vi "Center speed graph cursor on X.vi"(8 "error in (no error)":errorcluster) -> (0 "error out":errorcluster)   [LabVIEW 2020]
uses:
  Globals/gl_Time series viewer globals.vi
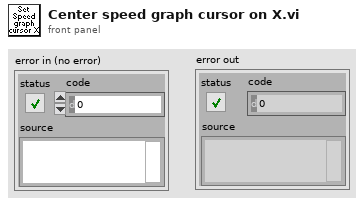
[diagram p1: front panel]
types:
  T1 = typedef "Time series viewer refs.ctl" = cluster{"This VI":refnum<vi>, "Image control":refnum<vi>, "AVI Mode ind":refnum<vi>, "Play":refnum<vi>, "Stop":refnum<vi>, "Back":refnum<vi>, "Scrollbar":refnum<vi>, "Video length info":refnum<vi>, "Expected speed values":refnum<vi>, "Intensity":refnum<vi>, "Path":refnum<vi>, "Selection sliders":refnum<vi>, "Speed Graph ref":refnum<vi>, "Frame rate set (fps)":refnum<vi>, "Number of rows to generate":refnum<vi>, "VL Image Array":refnum<vi>, "Image Scrollbar":refnum<vi>, "Channel to load":refnum<vi>, "Colour":refnum<vi>}
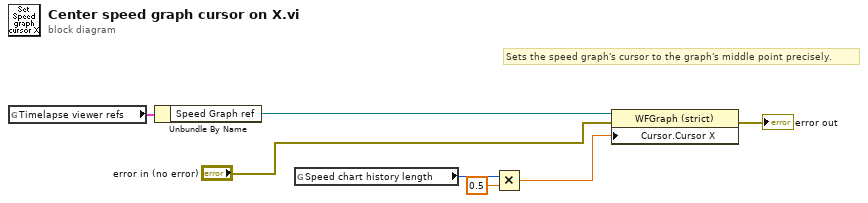
[diagram p0: block diagram]
diagram:
  # "Sets the speed graph's cursor to the graph's middle point precisely."
  n1 = global read "gl_Time series viewer globals.vi" "Timelapse viewer refs"() -> (w7:T1)
  n2 = Unbundle By Name(w7) -> ("Speed Graph ref"=w2:refnum<vi>)
  n3 = global read "gl_Time series viewer globals.vi" "Speed chart history length"() -> (w3:i32)
  n4 = Multiply(x=w3, y=0.5) -> (x*y=w5:dbl)
  n5 = property on="Property Node" class="WFGraph (strict)"(reference=w2, error in="error in (no error)", "Cursor.Cursor X"=w5) -> (error out=→"error out":errorcluster)  [unwired: 1 out]
